vi "Create.vi"(8 "error in (no error)":errorcluster, 10 "ID":string, 11 "Type":T1) -> (0 "error out":errorcluster, 3 "LVType out":refnum<class "LVType.lvclass">)   [LabVIEW 2020, in "LVDataTypes.lvlib" / "LVType.lvclass"]
uses:
  <vilib>/AppBuilder/Engine/WebServiceDescription/LVDataTypes/LVType/LVType.lvclass
  <vilib>/AppBuilder/Engine/WebServiceDescription/LVDataTypes/TypeCode.ctl
  <vilib>/AppBuilder/Engine/WebServiceDescription/LVDataTypes/LVType/LVType.lvclass/LVType.ctl
  <vilib>/AppBuilder/Engine/WebServiceDescription/LVDataTypes/LVDataTypes.lvlib
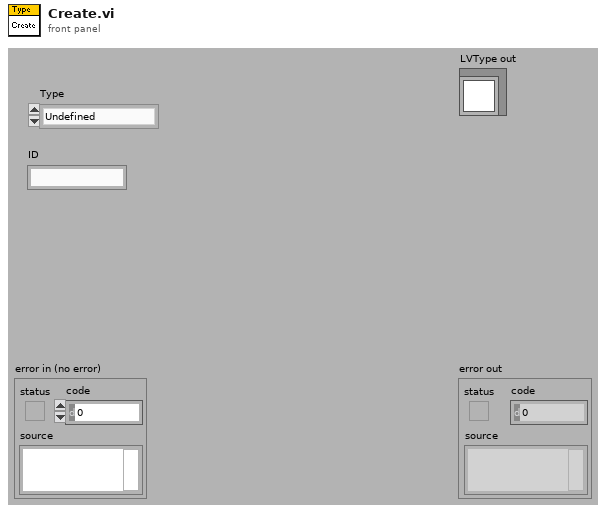
[diagram p1: front panel]
types:
  T1 = typedef "LVDataTypes.lvlib/TypeCode.ctl" = enum16{"Undefined", "Byte", "Unsigned Byte", "Word", "Unsigned Word", "Long", "Unsigned Long", "Quad", "Unsigned Quad", "Single", "Double", "Extended", "Enum", "Boolean", "String", "Path", "Array", "Cluster", "AnalogWaveform", "DigitalWaveform", "Time Stamp", "Void", "Complex Single", "Complex Double", "Complex Extended"}
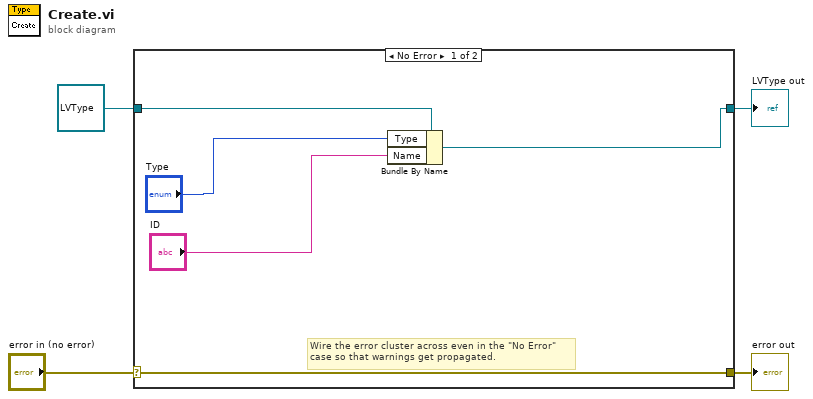
[diagram p0: block diagram]
diagram:
  n1 = case shown="No Error" "error in (no error)" {
    selector: "error in (no error)" -> [w9 w11]
    tunnel: [w9 w11] -> w3
    tunnel: [w6 w10] -> w1
    tunnel: refnum<class "LVType.lvclass"> refnum ("LVType in") -> [w7 w10]
    frame No Error {
      # "Wire the error cluster across even in the \"No Error\"\ncase so that warnings get propagated."
      n2 = Bundle By Name(cluster=w7, "Type"="Type", "Name"="ID") -> (w6:refnum<class "LVType.lvclass">)
    }
    frame Error {
    }
  }
  "error out" <- w3
  "LVType out" <- w1
